vi "oa_Build Waterfall Data Output.vi"(4 "windows info":cluster{"window type":u32, "window length":i32}={"window type"=62, "window length"=2048} {"window length" min=2; "window type" items=["None"=0, "Hanning"=1, "Hamming"=2, "Blackman-Harris"=3, "Exact Blackman"=4, "Blackman"=5, "Flat Top"=6, "4 Term B-Harris"=7, "7 Term B-Harris"=8, "Low Sidelobe"=9, "Gaussian"=62]}, 5 "reset? (F)":bool, 6 "plot type":T10(ring), 7 "dB on":bool, 9 "channel info":T7={"sensor sensitivity"=1000.0, "engineering units"=1, "dB reference"=1.0, "custom label"="EU", "weighting filter"=0, "pregain"=0.0} {"pregain" format="%.2f"; "weighting filter" items=["Linear", "A-weighting", "B-weighting", "C-weighting", "ITU-R 468-4", "Dolby", "CCITT", "C-message", "Wb", "Wc", "Wd", "We", "Wf", "Wh", "Wj", "Wk", "Wm", "AES17 20 kHz lowpass", "AES17 40 kHz lowpass", "AES17 20 kHz highpass", "AES17 40 kHz highpass"]; "dB reference" format="%^.1e"; "engineering units" items=["custom..."=0, "V"=1, "A"=21, "C"=30, "pC"=31, "s"=32, "-"=29, "Pa"=2, "N"=20, "g"=3, "m/s^2"=4, "m/s"=5, "m"=6, "mm/s"=12, "mm"=13, "micron/s"=14, "micron"=15, "in/s^2"=7, "in/s"=8, "in"=9, "mil/s"=10, "mil"=11, "rad/s^2"=16, "rad/s"=17, "rad"=18, "deg/s^2"=26, "deg/s"=27, "deg"=28, "RPM"=22, "cycle/s^2"=23, "Hz"=24, "cycle"=25, "strain"=19]; "sensor sensitivity" format="%#_5f"}, 10 "scales":T11 {"Y scale"."multiplier" format="%.2f"; "Y scale"."offset" format="%.2f"; "X scale"."multiplier" format="%.2f"; "X scale"."offset" format="%.2f"}, 11 "spectral map":dbl[][](array[numeric]) format="%.2f") -> (0 "spectrum info out":T1={"channel name"="", "description"="", "x-axis units"=0, "spectral info"={"spectrum type"=enum."Power [Magnitude^2]", "linear/dB"=enum."linear", "window"=0, "window size"=0, "FFT size"=0}, "engineering units"=0, "custom label"="", "dB reference [EU]"=0.0, "peak units"=enum."rms", "weighting filter"=0, "spectral density?"=FALSE, "unit label"="", "spectrum skewed?"=FALSE, "complimentary spectrum units"=enum."none"} {"x-axis units" items=["Time (s)"=0, "Frequency-CB (Hz)"=1, "Frequency-CPB (Hz)"=1248, "Frequency-Arbitrary (Hz)"=2357, "Quefrency (s)"=2, "Revolutions (rev)"=3, "Order"=4, "Speed (RPM)"=11, "Speed (rad/s)"=21, "Index"=65535]; "weighting filter" items=["Linear", "A-weighting", "B-weighting", "C-weighting", "ITU-R 468-4", "Dolby", "CCITT", "C-message", "Wb", "Wc", "Wd", "We", "Wf", "Wh", "Wj", "Wk", "Wm", "AES17 20 kHz lowpass", "AES17 40 kHz lowpass", "AES17 20 kHz highpass", "AES17 40 kHz highpass"]; "dB reference [EU]" format="%.2f"; "engineering units" items=["custom..."=0, "V"=1, "A"=21, "C"=30, "pC"=31, "s"=32, "-"=29, "Pa"=2, "N"=20, "g"=3, "m/s^2"=4, "m/s"=5, "m"=6, "mm/s"=12, "mm"=13, "micron/s"=14, "micron"=15, "in/s^2"=7, "in/s"=8, "in"=9, "mil/s"=10, "mil"=11, "rad/s^2"=16, "rad/s"=17, "rad"=18, "deg/s^2"=26, "deg/s"=27, "deg"=28, "RPM"=22, "cycle/s^2"=23, "Hz"=24, "cycle"=25, "strain"=19]; "spectral info"."window" items=["None "=0, "Hanning"=1, "Hamming"=2, "Blackman-Harris"=3, "Exact Blackman"=4, "Blackman"=5, "Flat Top"=6, "4 Term B-Harris "=7, "7 Term B-Harris"=8, "Low Sidelobe"=9, "Force - Exponential"=10, "Gaussian"=62]}, 1 "waterfall unit labels":T8, 3 "Waterfall Graph":T9)   [LabVIEW 2017, in "SoundVib_Resampling.lvlib"]
uses:
  <vilib>/addons/Sound and Vibration/Order Analysis/Resample Order Tracking/SoundVib_Resampling.lvlib
  <vilib>/addons/_NISVFA/_Shared subVIs/Controls/svc_Channel Info.ctl
  <vilib>/addons/_NISVFA/_Shared subVIs/Controls/svc_Engineering Units Text Ring.ctl
  <vilib>/addons/_NISVFA/_Shared subVIs/Controls/svc_Weighting Filter Text Ring.ctl
  <vilib>/addons/_NISVFA/_Shared subVIs/Controls/svc_Spectrum Info.ctl
  <vilib>/addons/_NISVFA/_Shared subVIs/Controls/svc_X-Axis Units.ctl
  <vilib>/addons/_NISVFA/_Shared subVIs/Controls/svc_Spectrum Type.ctl
  <vilib>/addons/_NISVFA/_Shared subVIs/Controls/svc_Complimentary Spectrum Units.ctl
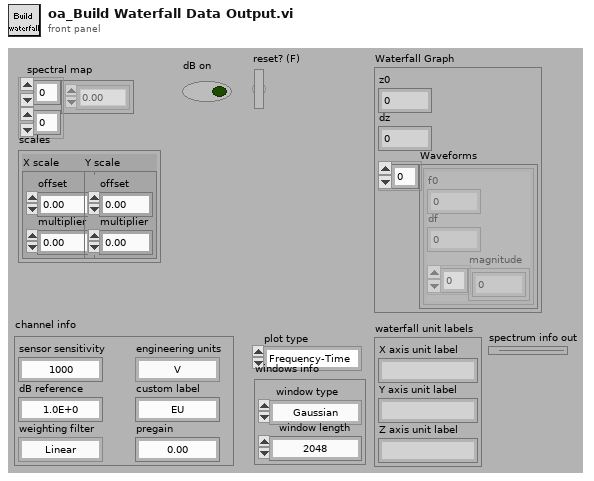
[diagram p1: front panel]
types:
  T1 = typedef "svc_Spectrum Info.ctl" = cluster{"channel name":string, "description":string, "x-axis units":T2, "spectral info":cluster{"spectrum type":T3, "linear/dB":enum16{"linear", "dB"}, "window":u16, "window size":i32, "FFT size":i32}, "engineering units":T4, "custom label":string, "dB reference [EU]":dbl, "peak units":enum16{"rms", "peak", "peak-peak"}, "weighting filter":T5, "spectral density?":bool, "unit label":string, "spectrum skewed?":bool, "complimentary spectrum units":T6}
  T2 = typedef "svc_X-Axis Units.ctl" = u16
  T3 = typedef "svc_Spectrum Type.ctl" = enum16{"FFT Spectrum [complex]", "Amplitude [Magnitude]", "Power [Magnitude^2]", "Cross Spectrum [complex]", "Frequency Response [Complex]"}
  T4 = typedef "svc_Engineering Units Text Ring.ctl" = u16
  T5 = typedef "svc_Weighting Filter Text Ring.ctl" = u16
  T6 = typedef "svc_Complimentary Spectrum Units.ctl" = enum16{"none", "radians", "degrees", "cycles", "imaginary"}
  T7 = typedef "svc_Channel Info.ctl" = cluster{"sensor sensitivity":dbl, "engineering units":T4, "dB reference":dbl, "custom label":string, "weighting filter":T5, "pregain":dbl}
  T8 = cluster{"X axis unit label":string, "Y axis unit label":string, "Z axis unit label":string}
  T9 = cluster{"z0":dbl, "dz":dbl, "Waveforms":cluster{"f0":dbl, "df":dbl, "magnitude":dbl[]}[]}
  T10 = enum16{"Frequency-Time", "Time-Frequency", "Order-Time", "Time-Order", "Frequency-RPM", "RPM-Frequency", "Order-RPM", "RPM-Order"}
  T11 = cluster{"X scale":cluster{"offset":dbl, "multiplier":dbl}, "Y scale":cluster{"offset":dbl, "multiplier":dbl}}
  T12 = cluster{"offset":dbl, "multiplier":dbl, "log view scaled signal":dbl[]}
  T13 = cluster{"offset":dbl, "multiplier":dbl, cluster{"offset":dbl, "multiplier":dbl, "log view scaled signal":dbl[]}[]}
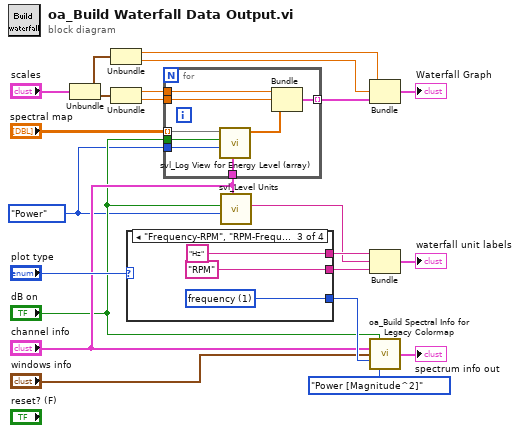
[diagram p0: block diagram]
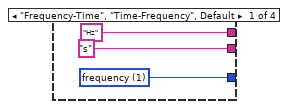
[diagram p2: hidden frame]
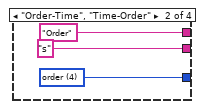
[diagram p3: hidden frame]
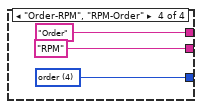
[diagram p4: hidden frame]
diagram:
  w1 = enum16{"Power", "Amplitude"}."Power" ("view mode")
  n1 = Unbundle("scales") -> ("X scale"=w16:cluster{"offset":dbl, "multiplier":dbl}, "Y scale"=w15:cluster{"offset":dbl, "multiplier":dbl})
  n2 = Unbundle(w16) -> ("offset"=w10:dbl, "multiplier"=w9:dbl)
  n3 = Unbundle(w15) -> ("offset"=w13:dbl, "multiplier"=w14:dbl)
  n4 = case shown="\"Frequency-RPM\", \"RPM-Frequency\"" "plot type" {
    tunnel: [w25 w28 w31 w34] -> w19
    tunnel: ["Hz" "Order" "Hz" "Order"] -> w6
    tunnel: ["s" "s" "RPM" "RPM"] -> w7
    frame "Frequency-Time", "Time-Frequency", Default {
      w25 = u16 1 items=["time"=0, "frequency"=1, "quefrency"=2, "revolutions"=3, "order"=4, "rpm"=11] ("x-axis units")
    }
    frame "Order-Time", "Time-Order" {
      w28 = u16 4 items=["time"=0, "frequency"=1, "quefrency"=2, "revolutions"=3, "order"=4, "rpm"=11] ("x-axis units")
    }
    frame "Frequency-RPM", "RPM-Frequency" {
      w31 = u16 1 items=["time"=0, "frequency"=1, "quefrency"=2, "revolutions"=3, "order"=4, "rpm"=11] ("x-axis units")
    }
    frame "Order-RPM", "RPM-Order" {
      w34 = u16 4 items=["time"=0, "frequency"=1, "quefrency"=2, "revolutions"=3, "order"=4, "rpm"=11] ("x-axis units")
    }
  }
  n5 = for {
    tunnel: [w42] -> w11 mode=indexing
    tunnel: w14 -> [w40]
    tunnel: w13 -> [w39]
    tunnel: "dB on" -> [w38]
    tunnel: "spectral map" -> [w37] mode=indexing
    tunnel: w1 -> [w36]
    tunnel: "channel info" -> [w35]
    n6 = call <vilib>:"svl_Log View for Energy Level (array).vi"("channel info"=w35, "view mode"=w36, "dB On (T)"=w38, "scaled signal"=w37) -> ("log view scaled signal"=w41:dbl[])  [unwired: 5 in, 2 out]
    n7 = Bundle("offset"=w39, "multiplier"=w40, "log view scaled signal"=w41) -> (w42:T12)  [unwired: 1 in]
  }
  n8 = call <vilib>:"svl_Level Units.vi"("channel info"="channel info", "view mode"=w1, "dB On (T)"="dB on") -> ("unit label"=w5:string)  [unwired: 6 in, 2 out]
  n9 = Bundle("offset"=w10, "multiplier"=w9, w11) -> (→"Waterfall Graph":T13)  [unwired: 1 in]
  n10 = Bundle(w6, "unit label"=w5, w7) -> (→"waterfall unit labels":cluster{string, "unit label":string, string})  [unwired: 1 in]
  n11 = call <vilib>:"oa_Build Spectral Info for Legacy Colormap.vi"("dB on (T)"="dB on", "channel info"="channel info", "windows info"="windows info", "x-axis units"=w19, "spectrum type"=svc_Spectrum_Type."Power [Magnitude^2]") -> ("spectrum info"=→"spectrum info out":T1)  [unwired: 9 in, 1 out]
